vi "Compile Channel Group Settings.vi"(8 "Channel Type":T1(ring), 9 "Group Name":string, 10 "ChannelSettings":T3, 11 "Group Settings":T2(array[cluster])) -> (3 "Group Settings":T2(array[cluster]))   [LabVIEW 2026, in "Template Deployment Hooks.lvlib"]
uses:
  Template Deployment Hooks.lvlib
  Shared/GroupedChannel.ctl
  Shared/GroupSettings.ctl
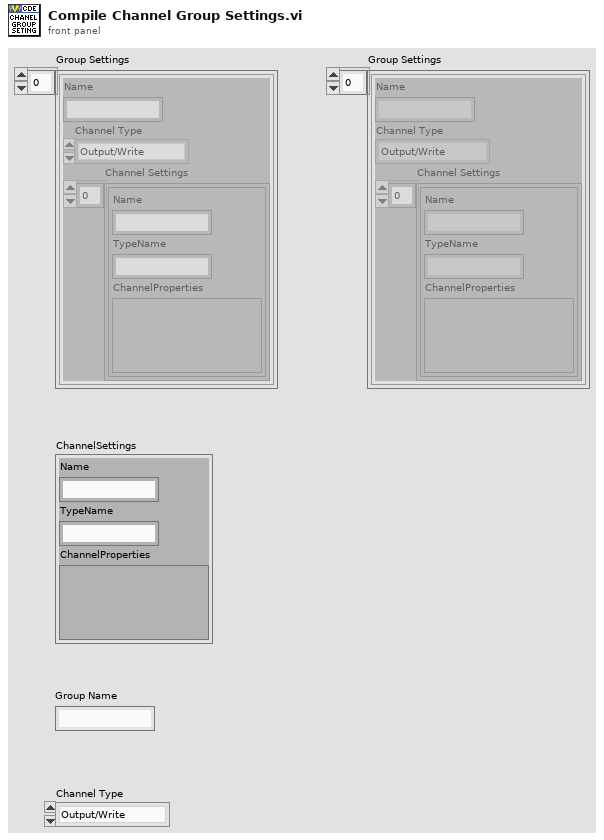
[diagram p1: front panel]
types:
  T1 = enum16{"Output/Write", "Input/Read", "Input/ReadWrite"}
  T2 = cluster{"Name":string, "Channel Type":enum16{"Output/Write", "Input/Read", "Input/ReadWrite"}, "Channel Settings":cluster{"Name":string, "TypeName":string, "ChannelProperties":variant}[]}[]
  T3 = cluster{"Name":string, "TypeName":string, "ChannelProperties":variant}
  T4 = typedef "GroupSettings.ctl" = cluster{"Name":string, "Channel Type":enum16{"Output/Write", "Input/Read", "Input/ReadWrite"}, "Channel Settings":T5[]}
  T5 = typedef "GroupedChannel.ctl" = cluster{"Name":string, "TypeName":string, "ChannelProperties":variant}
  T6 = cluster{"Name":string, "TypeName":string, "ChannelProperties":variant}[]
  T7 = cluster{"Name":string, "Channel Type":enum16{"Output/Write", "Input/Read", "Input/ReadWrite"}, "Channel Settings":cluster{"Name":string, "TypeName":string, "ChannelProperties":variant}[]}
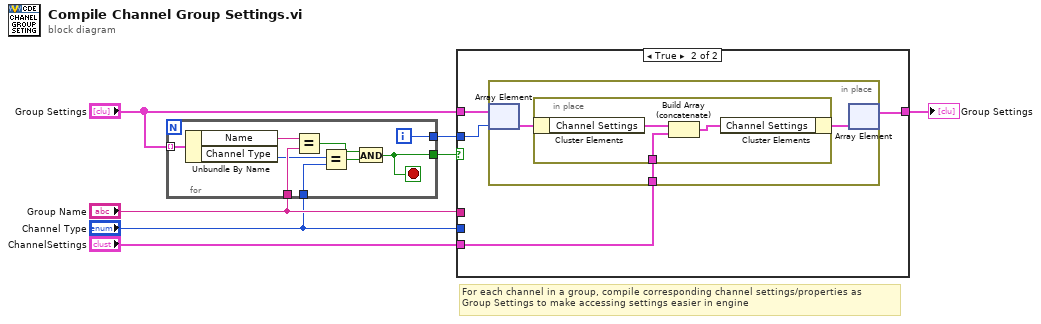
[diagram p0: block diagram]
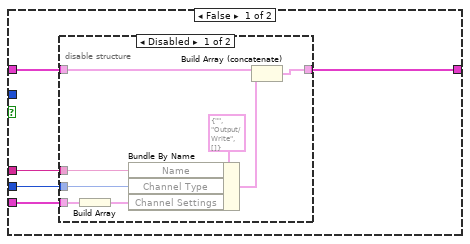
[diagram p2: hidden frame]
diagram:
  # "For each channel in a group, compile corresponding channel settings/properties as\nGroup Settings to make accessing settings easier in engine"
  n1 = for {
    tunnel: "Group Name" -> [w15]
    tunnel: [w12] -> w2
    tunnel: [w13] -> w1
    tunnel: "Group Settings" -> [w14] mode=indexing
    tunnel: "Channel Type" -> [w8]
    i -> [w13]
    stop <- w12 stop-if-true
    n2 = Unbundle By Name(w14) -> ("Name"=w16:string, "Channel Type"=w9:T1)
    n3 = Equal?(x=w16, y=w15) -> (x = y?=w11:bool)
    n4 = Equal?(x=w9, y=w8) -> (x = y?=w10:bool)
    n5 = And(x=w11, y=w10) -> (x .and. y?=w12:bool)
  }
  n6 = case shown="True" w2 {
    tunnel: [w18 w33] -> w6
    tunnel: "Group Settings" -> [w19 w34]
    tunnel: "ChannelSettings" -> [w20 w31]
    tunnel: w1 -> [_ w32]
    tunnel: "Group Name" -> [w21 _]
    tunnel: "Channel Type" -> [w17 _]
    frame False {
      n7 = disable-structure shown="Disabled" {
        disable-tunnel: w21 -> [w28 _]
        disable-tunnel: w20 -> [w27 _]
        disable-tunnel: w19 -> [w25 w30]
        disable-tunnel: [w23 w30] -> w18
        disable-tunnel: w17 -> [w22 _]
        frame Disabled {
          n8 = Build Array(w27) -> (w26:T6)
          n9 = Bundle By Name(cluster=T4 {"Name"="", "Channel Type"=enum."Output/Write", "Channel Settings"=[]} ("GroupSettings"), "Name"=w28, "Channel Type"=w22, "Channel Settings"=w26) -> (w24:T4)
          n10 = Build Array (concatenate)(w25, w24) -> (w23:T4[])
        }
        frame Enabled {
        }
      }
    }
    frame True {
      n11 = in-place {
        in-place-border: w31 -> [w35]
        n12 = in-place-array #1(w34, w32) -> (w37:T7)
        n13 = in-place {
          in-place-border: w35 -> [w39]
          n14 = in-place-cluster #2(w37) -> ("Channel Settings"=w40:T6)
          n15 = Build Array (concatenate)(w40, w39) -> (w38:T6)
          n16 = in-place-cluster #2("Channel Settings"=w38) -> (w36:T7)
        }
        n17 = in-place-array #1(w36) -> (w33:T2)  [unwired: 1 out]
      }
    }
  }
  "Group Settings" <- w6
